vi "Byte Array to I32.vi"(1 "Input Bytes":u8[](array[numeric]) format="%.0x") -> (0 "Output Integers":i32[](array[numeric]))   [LabVIEW 2025]
doc: "Changes unsigned array of bytes into 32 bit signed integers by combining bytes.\nScott Hannahs, NHMFL - FSU, Dec 1997\nAuthor: Scott Hannahs <sth@magnet.fsu.edu>\n\nThis software is licensed for use under the “MIT License\"\nCopyright (c) 2025 Scott Hannahs, sth@sth@magnet.sthnet.net\n\nPermission is hereby granted, free of charge, to any person obtaining a copy of this software and associated documentation files (the \"Software\"), to deal in the Software without restriction, including without limitation the rights to use, copy, modify, merge, publish, distribute, sublicense, and/or sell copies of the Software, and to permit persons to whom the Software is furnished to do so, subject to the following conditions: The above copyright notice and this permission notice shall be included in all copies or substantial portions of the Software.\n\nTHE SOFTWARE IS PROVIDED \"AS IS\", WITHOUT WARRANTY OF ANY KIND, EXPRESS OR IMPLIED, INCLUDING BUT NOT LIMITED TO THE WARRANTIES OF MERCHANTABILITY, FITNESS FOR A PARTICULAR PURPOSE AND NONINFRINGEMENT. IN NO EVENT SHALL THE AUTHORS OR COPYRIGHT HOLDERS BE LIABLE FOR ANY CLAIM, DAMAGES OR OTHER LIABILITY, WHETHER IN AN ACTION OF CONTRACT, TORT OR OTHERWISE, ARISING FROM, OUT OF OR IN CONNECTION WITH THE SOFTWARE OR THE USE OR OTHER DEALINGS IN THE SOFTWARE."
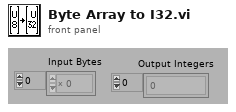
[diagram p1: front panel]
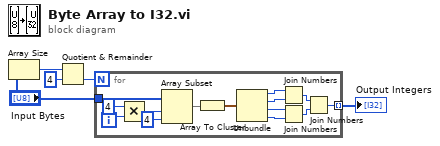
[diagram p0: block diagram]
diagram:
  n1 = Array Size(array="Input Bytes") -> (size(s)=w4:i32)
  n2 = Quotient & Remainder(x=w4, y=4) -> (floor(x/y)=w3:i32)  [unwired: 1 out]
  n3 = for {
    N: w3 -> [_]
    tunnel: [w17] -> w1 mode=indexing
    tunnel: "Input Bytes" -> [w12]
    i -> [w16]
    n4 = Multiply(x=4, y=w16) -> (x*y=w14:i32)
    n5 = Array Subset(array=w12, index=w14, length=4) -> (w11:u8[])
    n6 = Array To Cluster(array=w11) -> (cluster=w10:cluster{"[0]":u8, "[1]":u8, "[2]":u8, "[3]":u8})
    n7 = Unbundle(w10) -> ("[0]"=w9:u8, "[1]"=w8:u8, "[2]"=w7:u8, "[3]"=w6:u8)
    n8 = Join Numbers(hi=w9, lo=w8) -> ((hi.lo)=w19:u16)
    n9 = Join Numbers(hi=w7, lo=w6) -> ((hi.lo)=w18:u16)
    n10 = Join Numbers(hi=w19, lo=w18) -> ((hi.lo)=w17:u32)
  }
  "Output Integers" <- w1
